vi "UDP Refresh Estimated Array Size.vi"(8 "error in (no error)":errorcluster, 10 "UDP UI References in":T2, 11 "node References":T1) -> (0 "error out":errorcluster, 2 "UDP UI References out":T2, 3 "node References out":T1)   [LabVIEW 2015, in "E2E Tag Exchange editor node.lvclass"]
uses:
  E2E Tag Exchange editor node.lvclass
  UDP UI References.ctl
  object references.ctl
  <vilib>/NI/DCAF/Tag Editor Core/Configuration Editor/Classes/Engine Parent/Engine Parent Editor Node.lvclass
  <vilib>/NI/Tag Bus/tag/Data Type.ctl
  <vilib>/NI/Tag Bus Module Framework/channel/TBM channel.lvclass
  <vilib>/NI/Tag Bus/tag/tag descriptor.lvclass
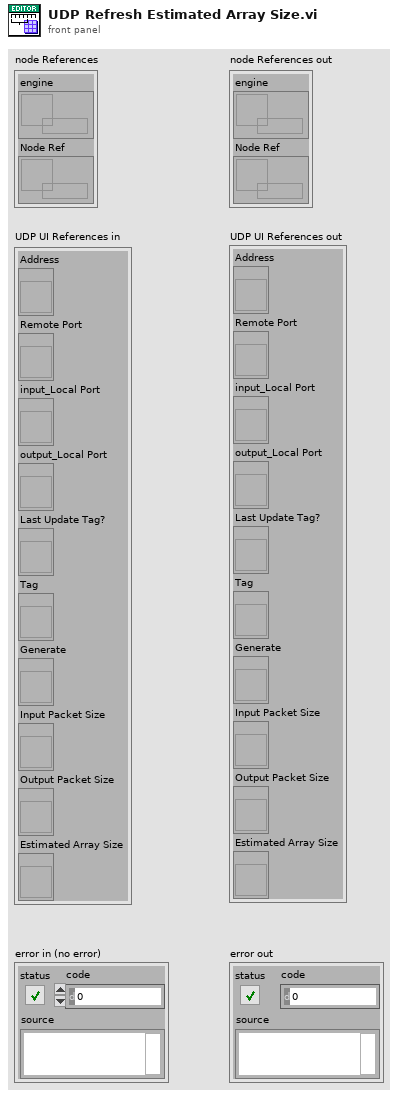
[diagram p1: front panel]
types:
  T1 = typedef "E2E Tag Exchange editor node.lvclass/object references.ctl" = cluster{"engine":refnum<data-value>, "Node Ref":refnum<data-value>}
  T2 = typedef "E2E Tag Exchange editor node.lvclass/UDP UI References.ctl" = cluster{"Address":refnum<vi>, "Remote Port":refnum<vi>, "input_Local Port":refnum<vi>, "output_Local Port":refnum<vi>, "Last Update Tag?":refnum<vi>, "Tag":refnum<vi>, "Generate":refnum<vi>, "Input Packet Size":refnum<vi>, "Output Packet Size":refnum<vi>, "Estimated Array Size":refnum<vi>}
  T3 = typedef "tag bus.lvlib/tag descriptor.lvclass/Data Type.ctl" = enum16{"Double", "Single", "I64", "I32", "I16", "I8", "U64", "U32", "U16", "U8", "Boolean", "String", "Array of Double", "Array of Single", "Array of I64", "Array of I32", "Array of I16", "Array of I8", "Array of U64", "Array of U32", "Array of U16", "Array of U8", "Array of Boolean", "Array of String"}
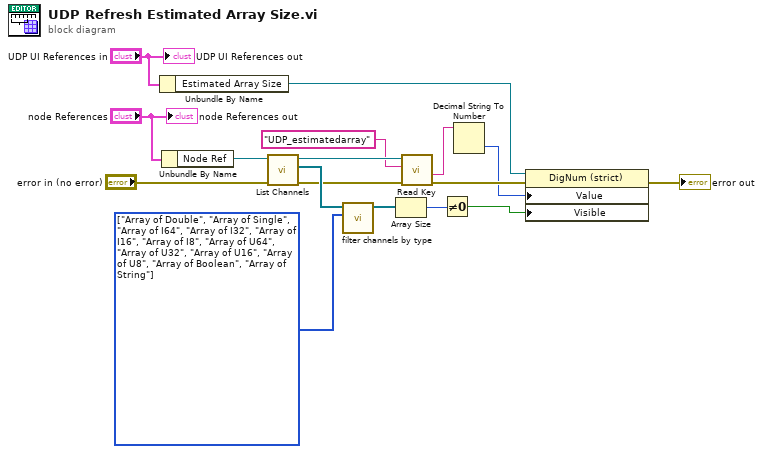
[diagram p0: block diagram]
diagram:
  w14 = T3[] [enum."Array of Double", enum."Array of Single", enum."Array of I64", enum."Array of I32", enum."Array of I16", enum."Array of I8", enum."Array of U64", enum."Array of U32", enum."Array of U16", enum."Array of U8", enum."Array of Boolean", enum."Array of String"] items=["Double", "Single", "I64", "I32", "I16", "I8", "U64", "U32", "U16", "U8", "Boolean", "String", "Array of Double", "Array of Single", "Array of I64", "Array of I32", "Array of I16", "Array of I8", "Array of U64", "Array of U32", "Array of U16", "Array of U8", "Array of Boolean", "Array of String"] ("allowed types")
  n1 = Unbundle By Name("UDP UI References in") -> ("Estimated Array Size"=w11:refnum<vi>)
  n2 = Unbundle By Name("node References") -> ("Node Ref"=w17:refnum<data-value>)
  n3 = call "List Channels.vi"("error in (no error)"="error in (no error)", "E2E editor node in"=w17) -> ("error out"=w6:errorcluster, "Input Channels"=w15:refnum<class "TBM channel.lvclass">[], "E2E editor node out"=w7:refnum<data-value>)  [unwired: 6 in, 1 out]
  n4 = call <vilib>:"filter channels by type.vi"("allowed types"=w14, "channels in"=w15) -> ("channels out"=w13:refnum<class "TBM channel.lvclass">[])  [unwired: 9 in]
  n5 = Array Size(array=w13) -> (size(s)=w12:i32)
  n6 = call "Read Key.vi"("error in (no error)"=w6, "Key"="UDP_estimatedarray", "E2E editor node in"=w7) -> ("error out"=w4:errorcluster, "Value"=w2:string)  [unwired: 6 in, 1 out]
  n7 = Not Equal To 0?(x=w12) -> (x != 0?=w3:bool)
  n8 = Decimal String To Number(string=w2) -> (number=w1:i32)  [unwired: 2 in, 1 out]
  n9 = property class="DigNum (strict)"(reference=w11, error in=w4, "Value"=w1, "Visible"=w3) -> (error out=→"error out":errorcluster)  [unwired: 1 out]
  "UDP UI References out" <- "UDP UI References in"
  "node References out" <- "node References"
